vi "DMM_Shutdown.vi"(3 "Input DMMP":refnum<class "DMMP.lvclass">) -> (0 "State":string="Baseline")   [LabVIEW 2014]
uses:
  DMMP.lvclass
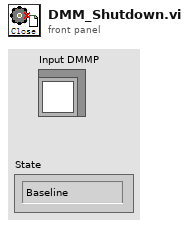
[diagram p1: front panel]
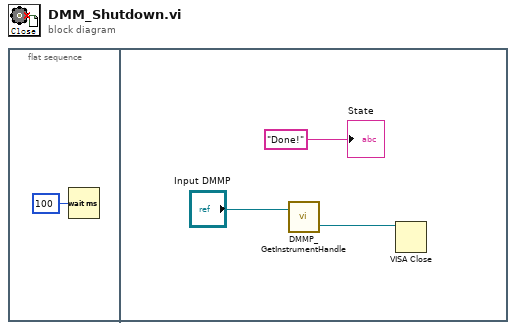
[diagram p0: block diagram]
diagram:
  n1 = flat-sequence {
    frame #0 {
      n2 = Wait (ms)(milliseconds to wait=u32 100) -> ()  [unwired: 1 out]
    }
    frame #1 {
      n3 = call "DMMP_GetInstrumentHandle.vi"("Input DMMP"="Input DMMP") -> ("DMM Serial Port"=w3:refnum<visa-resource-name>)  [unwired: 1 in, 1 out]
      n4 = VISA Close(VISA resource name=w3) -> ()  [unwired: 1 in, 1 out]
      "State" <- "Done!"
    }
  }
